vi "ReadValByNmString.vi"(5 "Type":string, 7 "Ctrl Name":string, 8 "error in":errorcluster caption="entrée d'erreur", 10 "CtrlRef":refnum<vi>[](array[refnum]), 11 "ControlsNames":string[](array[string])) -> (0 "error out":errorcluster caption="sortie d'erreur", 2 "Valeur":string, 3 "référence en sortie":refnum<vi>)   [LabVIEW 2019]
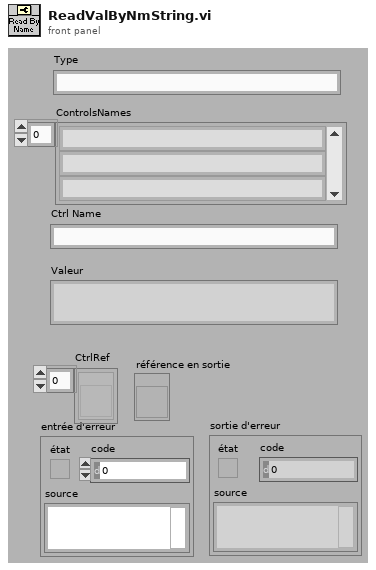
[diagram p1: front panel]
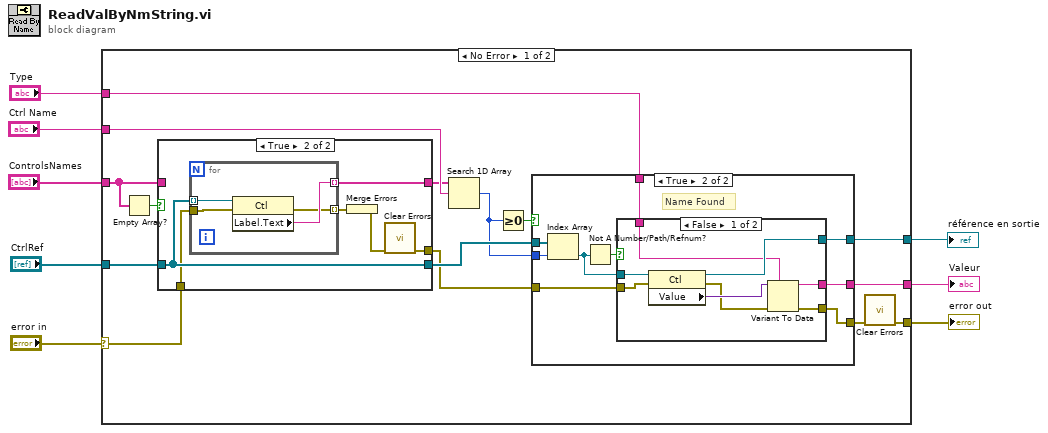
[diagram p0: block diagram]
diagram:
  n1 = case shown="No Error" "error in" {
    selector: "error in" -> [w13 w57]
    tunnel: [w23 _] -> w8
    tunnel: [w10 w57] -> w6
    tunnel: "ControlsNames" -> [w14 _]
    tunnel: "Ctrl Name" -> [w17 _]
    tunnel: "CtrlRef" -> [w18 _]
    tunnel: [w21 _] -> w2
    tunnel: "Type" -> [w12 _]
    frame No Error {
      n2 = Empty Array?(array=w14) -> (empty?=w20:bool)
      n3 = case shown="True" w20 {
        tunnel: [w26 w32] -> w19
        tunnel: w18 -> [w26 w32]
        tunnel: [w25 w31] -> w15
        tunnel: w14 -> [w25 _]
        tunnel: w13 -> [w24 w30]
        tunnel: [w24 w27] -> w11
        frame False {
        }
        frame True {
          n4 = for {
            tunnel: w32 -> [w36] mode=indexing
            tunnel: [w35] -> w31 mode=indexing
            tunnel: w30 -> [w34]
            tunnel: [w33] -> w29 mode=indexing
            n5 = property class="Ctl"(reference=w36, error in=w34) -> (error out=w33:errorcluster, "Label.Text"=w35:string)  [unwired: 1 out]
          }
          n6 = Merge Errors(w29) -> (w28:errorcluster)
          n7 = call <vilib>:"Clear Errors.vi"("error in (no error)"=w28) -> ("error out"=w27:errorcluster)  [unwired: 5 in, 1 out]
        }
      }
      n8 = Search 1D Array(1D array=w15, element=w17) -> (index of element=w16:i32)  [unwired: 1 in]
      n9 = Greater Or Equal To 0?(x=w16) -> (x >= 0?=w22:bool)
      n10 = case shown="True" w22 {
        tunnel: [_ w45] -> w23
        tunnel: w19 -> [_ w44]
        tunnel: w16 -> [_ w43]
        tunnel: [_ w41] -> w21
        tunnel: w12 -> [_ w40]
        tunnel: w11 -> [w37 w39]
        tunnel: [w37 w38] -> w9
        frame False {
          # "Name Not Found"
        }
        frame True {
          # "Name Found"
          n11 = Index Array(array=w44, index=w43) -> (element=w42:refnum<vi>)
          n12 = Not A Number/Path/Refnum?(number/path/refnum=w42) -> (NaN/Path/Refnum?=w46:bool)
          n13 = case shown="False" w46 {
            tunnel: w42 -> [w53 w56]
            tunnel: [w50 _] -> w45
            tunnel: [w54 w56] -> w41
            tunnel: w40 -> [w51 _]
            tunnel: w39 -> [w49 w55]
            tunnel: [w47 w55] -> w38
            frame False {
              n14 = property class="Ctl"(reference=w53, error in=w49) -> (reference out=w54:refnum<vi>, error out=w48:errorcluster, "Value"=w52:variant)
              n15 = Variant To Data(error in=w48, type=w51, Variant=w52) -> (data=w50:string, error out=w47:errorcluster)
            }
            frame True {
              # "Invalid Ref"
            }
          }
        }
      }
      n16 = call <vilib>:"Clear Errors.vi"("error in (no error)"=w9) -> ("error out"=w10:errorcluster)  [unwired: 5 in, 1 out]
    }
    frame Error {
    }
  }
  "Valeur" <- w8
  "error out" <- w6
  "référence en sortie" <- w2
